vi "Power Spectrum PtByPt.vi"(2 "initialize":bool, 3 "sample length":i32=100, 5 "x":dbl format="%0.2f") -> (0 "error":i32, 1 "Power Spectrum":dbl[](array[numeric]))   [LabVIEW 2020, in "NI_PtbyPt.lvlib"]
doc: "Computes the <B>Power Spectrum</B>, Sxx, of the set of input data points specified by <B>sample length</B>."
uses:
  <vilib>/ptbypt/NI_PtbyPt.lvlib
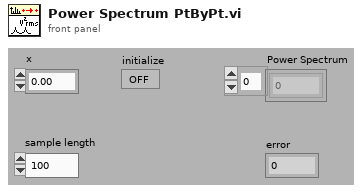
[diagram p1: front panel]
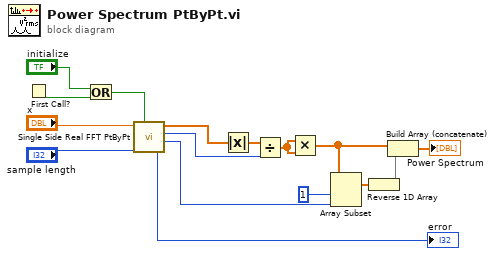
[diagram p0: block diagram]
diagram:
  n1 = First Call?() -> (First Call?: T/F=w1:bool)
  n2 = Or(x="initialize", y=w1) -> (x .or. y?=w2:bool)
  n3 = call <vilib>:"Single Side Real FFT PtByPt.vi"("initialize"=w2, "sample length"="sample length", "input data"="x") -> ("error"=→"error":i32, "half length"=w6:i32, "sample length"=w5:i32, "FFT Single Side"=w4:cdb[])  [unwired: 2 in]
  n4 = Absolute Value(x=w4) -> (abs(x)=w14:dbl[])
  n5 = Divide(x=w14, y=w5) -> (x/y=w12:dbl[])
  n6 = Multiply(x=w12, y=w12) -> (x*y=w13:dbl[])
  n7 = Array Subset(array=w13, index=1 ("Array Index"), length=w6) -> (w15:dbl[])
  n8 = Reverse 1D Array(array=w15) -> (reversed array=w11:dbl[])
  n9 = Build Array (concatenate)(w13, w11) -> (→"Power Spectrum":dbl[])
